vi "simpleCode2.vi"() -> ()   [LabVIEW 2020]
panel:
  out "inner i":i32
  out "outer i":i32
  out "inner out":i32
  in  "inner":i32
  in  "outer":i32
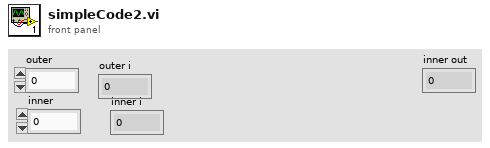
[diagram p1: front panel]
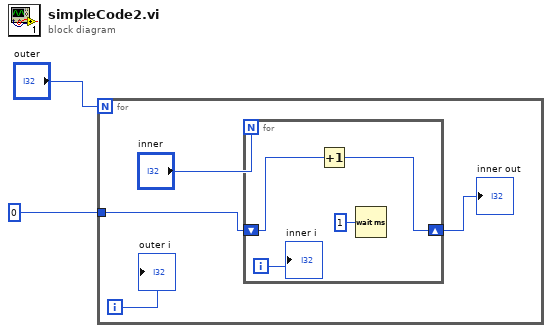
[diagram p0: block diagram]
diagram:
  n1 = for {
    N: "outer" -> [_]
    tunnel: 0 -> [w3]
    i -> [w4]
    n2 = for {
      N: "inner" -> [_]
      shift-right: [w9] -> w5
      shift-left: w3 -> [w10]
      i -> [w7]
      n3 = Increment(x=w10) -> (x+1=w9:i32)
      n4 = Wait (ms)(milliseconds to wait=u32 1) -> ()  [unwired: 1 out]
      "inner i" <- w7
    }
    "inner out" <- w5
    "outer i" <- w4
  }
